vi "test_signal2word.vi"() -> ()   [LabVIEW 2020]
uses:
  Source/RT Driver/RT Driver/Controls/Asynchronous - Parameter map_type.ctl
  Source/Shared/EncodeDecode/_typedefs/parameter_config_type.ctl
  Source/Shared/EncodeDecode/_typedefs/parameter_config_type_type.ctl
  Source/Shared/EncodeDecode/_typedefs/parameter_config_encoding_type.ctl
  Source/RT Driver/Ballard MIL-1553 Engine.lvlib
panel:
  out "words out":u16[](array[numeric]) format="%016b"
  in  "parameters in":dbl[](array[numeric])
  in  "param map":T1
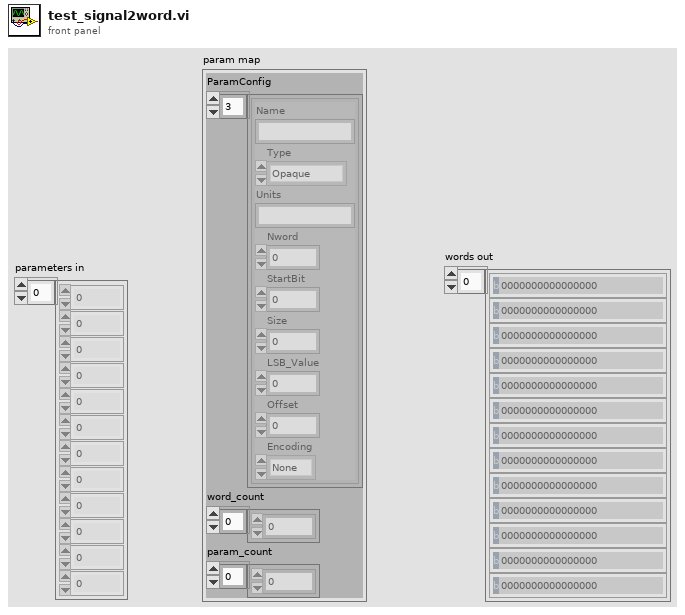
[diagram p1: front panel]
types:
  T1 = typedef "Ballard MIL-1553 Engine.lvlib/Asynchronous - Parameter map_type.ctl" = cluster{"ParamConfig":T2[], "word_count":u8[], "param_count":u8[]}
  T2 = typedef "parameter_config_type.ctl" = cluster{"Name":string, "Type":T3, "Units":string, "Nword":i32, "StartBit":i32, "Size":i32, "LSB_Value":i32, "Offset":i32, "Encoding":T4}
  T3 = typedef "parameter_config_type_type.ctl" = enum16{"Opaque", "Enum", "Float", "Integer", "Bcd", "Bool"}
  T4 = typedef "parameter_config_encoding_type.ctl" = enum16{"None", "2-complement", "Unsigned"}
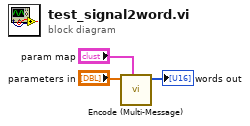
[diagram p0: block diagram]
diagram:
  n1 = call "Encode (Multi-Message).vi"("param map"="param map", "parameters in"="parameters in") -> ("words out"=→"words out":u16[])  [unwired: 9 in]
